vi "CODMn启动 (子VI).vi"(9 "强制切换":bool, 10 "CODMn量程切换":enum32{"H", "L", "AUTO"}(ring)=enum."AUTO", 11 "启动测量模式":T2) -> (0 "error out":T1={"status"=FALSE, "代码"=4, "source"=""} caption="错误输出" {"代码" items=["执行成功"=1, "执行失败，但不知道原因"=2, "命令请求条件错误"=3, "通讯超时"=4, "系统繁忙不能执行"=5, "系统故障"=6, "没有数据"=100]})   [LabVIEW 2016]
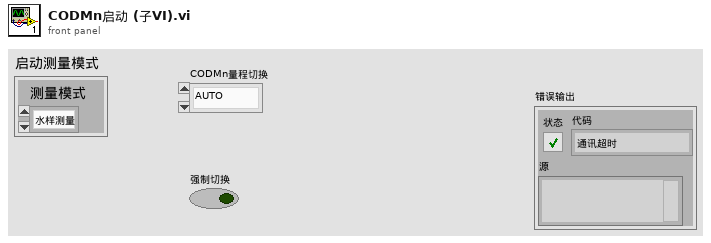
[diagram p1: front panel]
types:
  T1 = cluster{"status":bool, "代码":u16, "source":string}
  T2 = cluster{"测量模式":enum16{"水样测量", "标样核查", "零点核查", "跨度核查", "空白测试", "加标回收", "平行样", "校零", "校标"}}
  T3 = enum16{"空闲", "水样测试", "标样核查", "零点核查", "跨度核查", "空白测试", "平行样测试", "质控样", "空白校准", "标样校准", "加标回收"}
  T4 = cluster{"命令":string, "测量模式":enum16{"水样测量", "标样核查", "零点核查", "跨度核查", "空白测试", "加标回收", "平行样", "校零", "校标"}, "CODMn量程切换":enum32{"H", "L", "AUTO"}}
  T5 = enum16{"水样测量", "标样核查", "零点核查", "跨度核查", "空白测试", "加标回收", "平行样", "校零", "校标"}
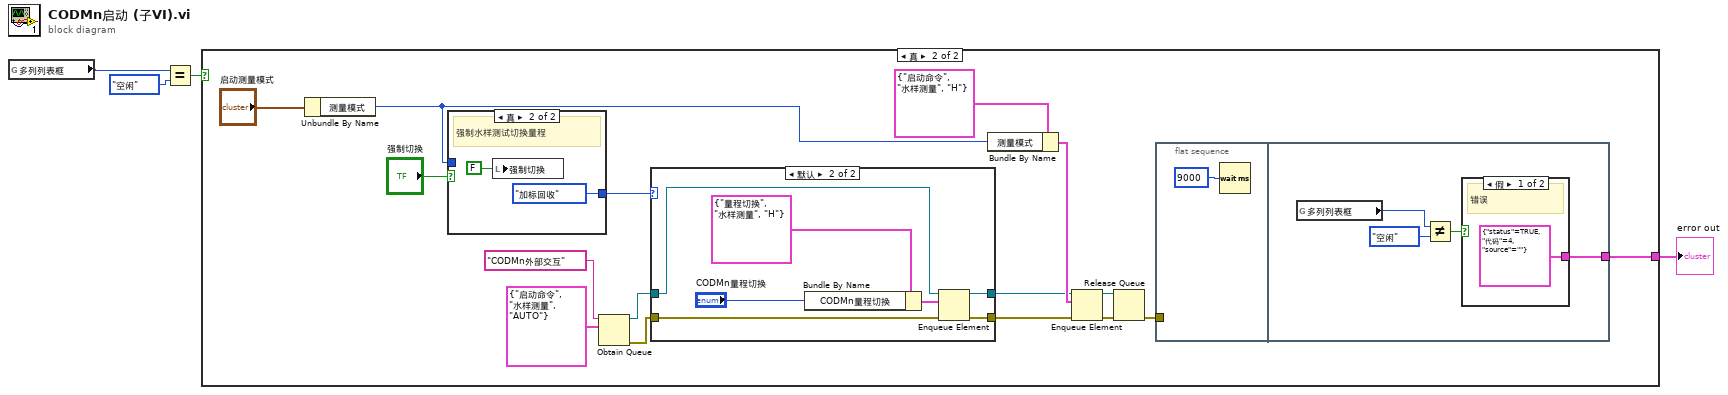
[diagram p0: block diagram]
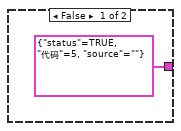
[diagram p2: hidden frame]
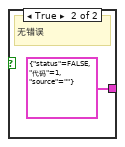
[diagram p3: hidden frame]
diagram:
  n1 = global read "运行时序全局变量.vi" "多列列表框"() -> (w1:i32)
  n2 = Equal?(x=w1, y=T3."空闲") -> (x = y?=w3:bool)
  n3 = case shown="真" w3 {
    tunnel: [T1 {"status"=TRUE, "代码"=5, "source"=""} ("error out") w6] -> w2
    frame False {
    }
    frame True {
      n4 = Unbundle By Name("启动测量模式") -> ("测量模式"=w9:T5)
      n5 = case shown="真" "强制切换" {
        tunnel: w9 -> [w29 _]
        tunnel: [w29 T5."加标回收" ("测量模式")] -> w8
        frame False {
        }
        frame True {
          # "强制水样测试切换量程"
          n6 = local write "强制切换"(FALSE ("强制切换")) -> ()
        }
      }
      n7 = Obtain Queue(name (unnamed)="CODMn外部交互" ("名称（未命名）"), element data type=T4 {"命令"="启动命令", "测量模式"=enum."水样测量", "CODMn量程切换"=enum."AUTO"} ("元素")) -> (queue out=w14:refnum<queue>, error out=w13:errorcluster)  [unwired: 3 in, 1 out]
      n8 = case shown="默认" w8 {
        tunnel: w14 -> [w33 w40]
        tunnel: w13 -> [w32 w39]
        tunnel: [w33 w38] -> w12
        tunnel: [w32 w37] -> w11
        frame "水样测量" {
        }
        frame Default {
          n9 = Bundle By Name(cluster=T4 {"命令"="量程切换", "测量模式"=enum."水样测量", "CODMn量程切换"=enum."H"} ("元素"), "CODMn量程切换"="CODMn量程切换") -> (w35:T4)
          n10 = Enqueue Element(queue=w40, element=w35, error in (no error)=w39) -> (queue out=w38:refnum<queue>, error out=w37:errorcluster)  [unwired: 1 in, 1 out]
        }
      }
      n11 = Bundle By Name(cluster=T4 {"命令"="启动命令", "测量模式"=enum."水样测量", "CODMn量程切换"=enum."H"} ("元素"), "测量模式"=w9) -> (w15:T4)
      n12 = Enqueue Element(queue=w12, element=w15, error in (no error)=w11) -> (queue out=w19:refnum<queue>, error out=w18:errorcluster)  [unwired: 1 in, 1 out]
      n13 = Release Queue(queue=w19, error in (no error)=w18) -> (error out=w7:errorcluster)  [unwired: 1 in, 2 out]
      n14 = flat-sequence {
        tunnel: w7 -> [_]
        tunnel: [w24] -> w6
        frame #0 {
          n15 = Wait (ms)(milliseconds to wait=u32 9000 ("等待时间（毫秒）")) -> ()  [unwired: 1 out]
        }
        frame #1 {
          n16 = global read "运行时序全局变量.vi" "多列列表框"() -> (w23:i32)
          n17 = Not Equal?(x=w23, y=T3."空闲") -> (x != y?=w25:bool)
          n18 = case shown="假" w25 {
            tunnel: [T1 {"status"=TRUE, "代码"=4, "source"=""} ("error out") T1 {"status"=FALSE, "代码"=1, "source"=""} ("error out")] -> w24
            frame False {
              # "错误"
            }
            frame True {
              # "无错误"
            }
          }
        }
      }
    }
  }
  "error out" <- w2
